vi "Config BERT Display.vi"(8 "error in (no error)":errorcluster {"code" format="%.0x"}, 9 "Display Update (F:CONTINUOUS)":bool, 10 "Display BER (T:%)":bool=TRUE, 11 "VISA Resource Name":refnum<visa-resource-name>) -> (0 "error out":errorcluster {"code" format="%.0x"}, 3 "VISA Resource Name Out":refnum<visa-resource-name>)   [LabVIEW 2012, in "Agilent ESG Series.lvlib"]
doc: "This VI is used to configure the parameters associated with the display of the BER test measurements."
uses:
  <instrlib>/Agilent ESG Series/Agilent ESG Series.lvlib
panel:
  # "%"
  # "EXP"
  # "CYCLE END"
  # "CONTINUOUS"
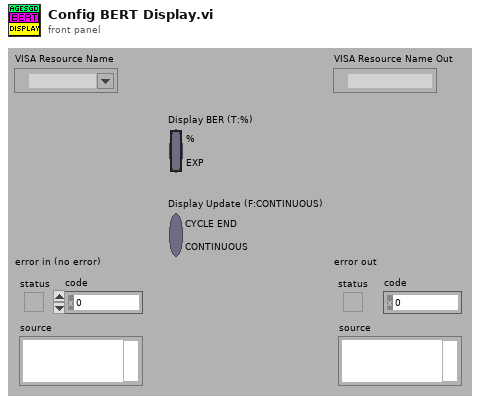
[diagram p1: front panel]
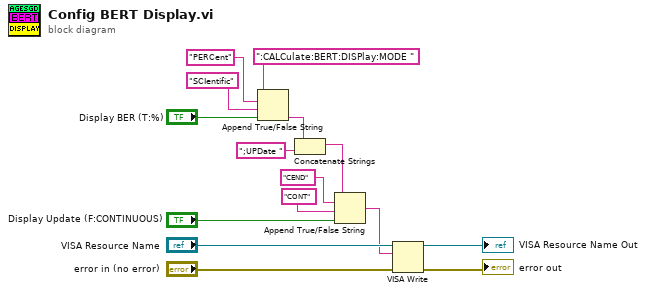
[diagram p0: block diagram]
diagram:
  n1 = Append True/False String(1:"Display BER (T:%)", 2:"SCIentific" ("false string"), 3:"PERCent" ("true string"), 4:":CALCulate:BERT:DISPlay:MODE " ("string (\"\")")) -> (0:w9:string)
  n2 = Concatenate Strings(w9, ";UPDate ") -> (w5:string)
  n3 = Append True/False String(1:"Display Update (F:CONTINUOUS)", 2:"CONT" ("false string"), 3:"CEND" ("true string"), 4:w5) -> (0:w1:string)
  n4 = VISA Write(VISA resource name="VISA Resource Name", write buffer=w1, error in (no error)="error in (no error)") -> (VISA resource name out=→"VISA Resource Name Out":refnum<visa-resource-name>, error out=→"error out":errorcluster)  [unwired: 1 out]
